vi "Player Info.vi"(11 "Snail In":refnum<class "Cautious Random Location.lvclass">) -> (1 "Victory Speech":string, 2 "Name":string, 3 "Snail Out":refnum<class "Cautious Random Location.lvclass">)   [LabVIEW 2015, in "Cautious Random Location.lvclass"]
uses:
  Cautious Random Location.lvclass
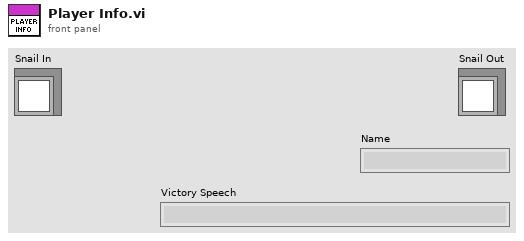
[diagram p1: front panel]
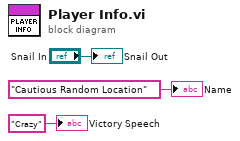
[diagram p0: block diagram]
diagram:
  "Snail Out" <- "Snail In"
  "Name" <- "Cautious Random Location" ("Name")
  "Victory Speech" <- "Crazy" ("Victory Speech")
